vi "Write charset.vi"(8 "error in (no error)":errorcluster, 10 "charset":u8[](array[numeric]), 11 "Serializer.Base64 in":refnum<class "Serializer.Base64.lvclass">) -> (0 "error out":errorcluster, 3 "Serializer.Base64 out":refnum<class "Serializer.Base64.lvclass">)   [LabVIEW 2013, in "Serializer.Base64.lvclass"]
uses:
  Serializer.Base64.lvclass
  Serializer.Base64.lvclass/Serializer.Base64.ctl
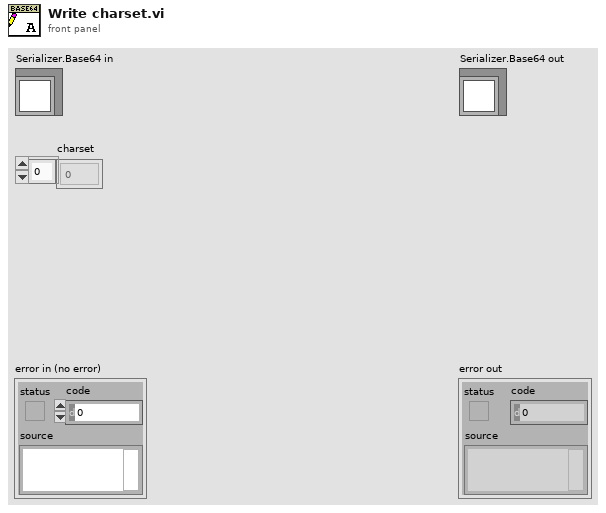
[diagram p1: front panel]
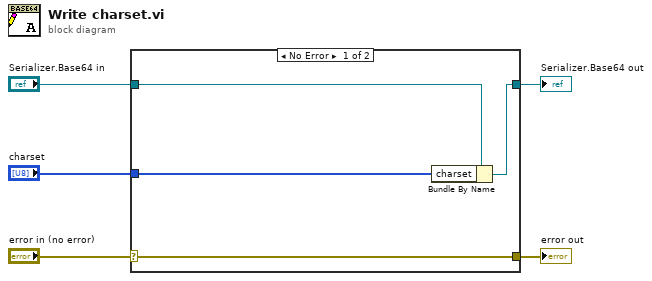
[diagram p0: block diagram]
diagram:
  n1 = case shown="No Error" "error in (no error)" {
    selector: "error in (no error)" -> [w9 w10]
    tunnel: [w9 w10] -> w4
    tunnel: [w7 w11] -> w2
    tunnel: "Serializer.Base64 in" -> [w8 w11]
    tunnel: "charset" -> [w6 _]
    frame No Error {
      n2 = Bundle By Name(cluster=w8, "charset"=w6) -> (w7:refnum<class "Serializer.Base64.lvclass">)
    }
    frame Error {
    }
  }
  "error out" <- w4
  "Serializer.Base64 out" <- w2
